vi "setSortOptions.vi"(8 "error in (no error)":errorcluster, 10 "SortOptions":T1, 11 "BasicSortedList in":refnum<class "BasicSortedList.lvclass">) -> (0 "error out":errorcluster, 3 "BasicSortedList out":refnum<class "BasicSortedList.lvclass">)   [LabVIEW 2010, in "BasicSortedList.lvclass"]
doc: "Set if the sorted list is asceding or decending."
uses:
  BasicSortedList.lvclass
  BasicSortOptions.ctl
  BasicSortedList.lvclass/BasicSortedList.ctl
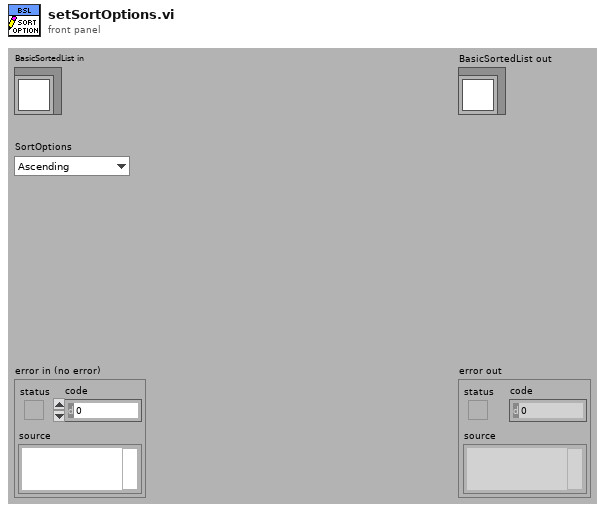
[diagram p1: front panel]
types:
  T1 = typedef "BasicSortedList.lvclass/BasicSortOptions.ctl" = enum16{"Ascending", "Decending"}
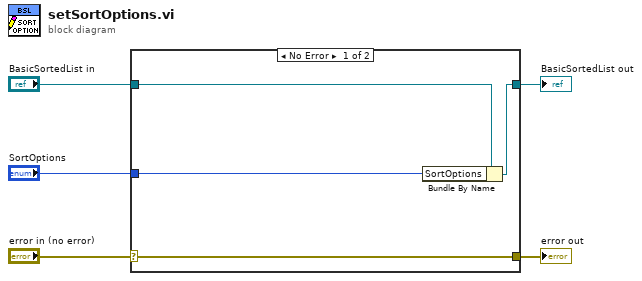
[diagram p0: block diagram]
diagram:
  n1 = case shown="No Error" "error in (no error)" {
    selector: "error in (no error)" -> [w9 w10]
    tunnel: [w9 w10] -> w4
    tunnel: [w7 w11] -> w2
    tunnel: "BasicSortedList in" -> [w8 w11]
    tunnel: "SortOptions" -> [w6 _]
    frame No Error {
      n2 = Bundle By Name(cluster=w8, "SortOptions"=w6) -> (w7:refnum<class "BasicSortedList.lvclass">)
    }
    frame Error {
    }
  }
  "error out" <- w4
  "BasicSortedList out" <- w2
